vi "DWF Dig Write.vi"(0 "Instrument Handle In":u32, 5 "Lines":string, 7 "Data":bool[](array[boolean]), 11 "Error In":errorcluster caption="Error In (no error)") -> (4 "Instrument Handle Out":u32, 15 "Error Out":errorcluster)   [LabVIEW 2015, in "DigilentWF.lvlib"]
doc: "Writes data to the specified lines."
uses:
  <vilib>/DigilentWF/DigilentWF.lvlib
  dwf.dll
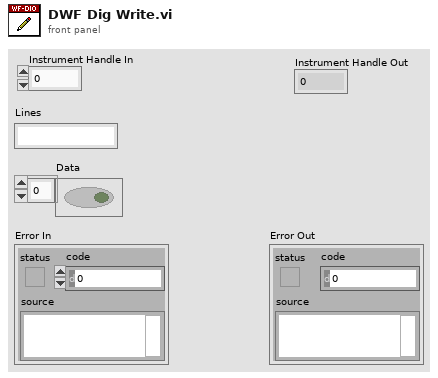
[diagram p1: front panel]
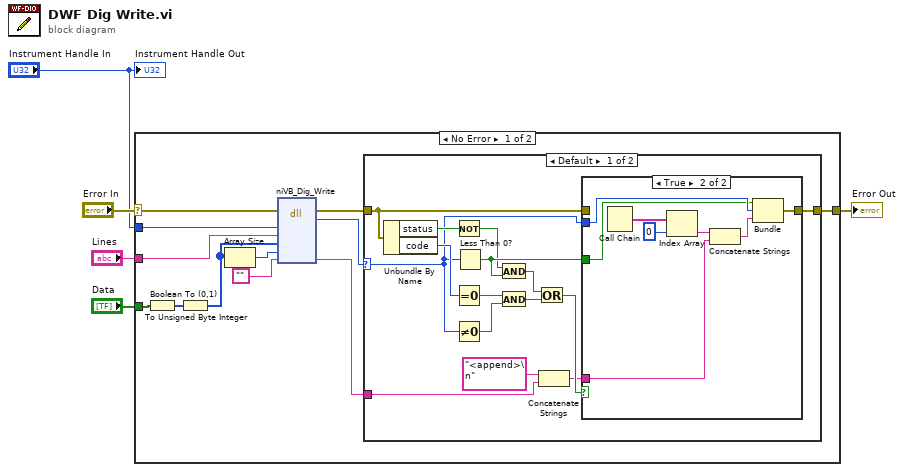
[diagram p0: block diagram]
diagram:
  n1 = case "outter_case" shown="No Error" "Error In" {
    selector: "Error In" -> [w13 w43]
    tunnel: [w17 w43] -> w4
    tunnel: "Instrument Handle In" -> [w12 _]
    tunnel: "Lines" -> [w15 _]
    tunnel: "Data" -> [w16 _]
    frame No Error {
      n2 = Boolean To (0,1)(Boolean=w16) -> (0, 1=w11:i16[])
      n3 = To Unsigned Byte Integer(number=w11) -> (unsigned 8bit integer=w8:u8[])
      n4 = Array Size(array=w8) -> (size(s)=w10:i32)
      n5 = dll-call lib="dwf.*" fn="niVB_Dig_Write"(error in=w13, "instrumentHandle"=w12, "lines"=w15, "data"=w8, "dataSize"=w10, "szError"="") -> (error out=w14:errorcluster, "return type"=w9:i32, "szError"=w7:string)  [unwired: 6 in, 1 out]
      n6 = case "inner_case" shown="Default" w9 {
        selector: w9 -> [w22 _]
        tunnel: w14 -> [w23 w42]
        tunnel: [w19 w42] -> w17
        tunnel: w7 -> [w18 _]
        frame Default {
          n7 = Unbundle By Name(w23) -> ("status"=w27:bool, "code"=w31:i32)
          n8 = Not(x=w27) -> (.not. x?=w30:bool)
          n9 = Equal To 0?(x=w31) -> (x = 0?=w26:bool)
          n10 = Not Equal To 0?(x=w22) -> (x != 0?=w29:bool)
          n11 = Less Than 0?(x=w22) -> (x < 0?=w32:bool)
          n12 = And(x=w30, y=w32) -> (x .and. y?=w28:bool)
          n13 = And(x=w26, y=w29) -> (x .and. y?=w25:bool)
          n14 = Or(x=w28, y=w25) -> (x .or. y?=w24:bool)
          n15 = Concatenate Strings("<append>\n" ("string"), w18) -> (w21:string)
          n16 = case shown="True" w24 {
            tunnel: [w33 w40] -> w19
            tunnel: w22 -> [_ w39]
            tunnel: w32 -> [_ w38]
            tunnel: w23 -> [w33 _]
            tunnel: w21 -> [_ w34]
            frame False {
            }
            frame True {
              n17 = Call Chain() -> (call chain=w37:string[])
              n18 = Index Array(array=w37, index=0) -> (element=w36:string)
              n19 = Concatenate Strings(w36, w34) -> (w41:string)
              n20 = Bundle(w38, "return type"=w39, w41) -> (w40:cluster{bool, "return type":i32, string})  [unwired: 1 out]
            }
          }
        }
        frame 0 {
        }
      }
    }
    frame Error {
    }
  }
  "Error Out" <- w4
  "Instrument Handle Out" <- "Instrument Handle In"
